vi "UpdateCtrlParams.vi"(6 "Ignore Update? (F)":bool, 8 "error in (no error)":errorcluster, 9 "Ts [s]":dbl caption="FPGA Ctrl Loop \nTime (Ts) [s]", 10 "Controller Gains":T2={"Z-direction"={"Kp"=1.0, "Ki"=50.0, "fLPF"=0.0}, "ThX-direction"={"Kp"=1.0, "Ki"=0.0, "fLPF"=0.0}, "ThY-direction"={"Kp"=1.0, "Ki"=0.0, "fLPF"=0.0}, "Bow-direction"={"Kp"=1.0, "Ki"=0.0, "fLPF"=0.0}, "Tor-direction"={"Kp"=0.0, "Ki"=0.0, "fLPF"=0.0}}, 11 "FPGA VI Reference In":T1) -> (0 "error out":errorcluster, 3 "FPGA VI ReferenceOut":T1)   [LabVIEW 2020, in "FPGAcontrolIO.lvlib"]
doc: "Update FPGA controller parameters"
uses:
  FPGAcontrolIO.lvlib
  PC/Controller/TypeDefs/ControllerGains_UI.ctl
  PC/Controller/TypeDefs/ControllerGains_IndAxis.ctl
  FPGA/Components/FPGA TypeDefs/FPGA_Ref_TypeDef.ctl
  PC/Components/Controller/TypeDefs/LPF params.ctl
  <vilib>/Utility/error.llb/Error Cluster From Error Code.vi
  <vilib>/rvi/errors/niLvFpgaAdjustHostInterfaceError.vi
  <vilib>/rvi/interface/nirviReadWriteControl/nirviReadWriteControl.xnode
  PC/Components/Controller/PC-RT_Controller.lvlib
  NiFpgaLv.dll
  <vilib>/rvi/interface/Simulation/niFpgaSimulationCallBeginRW.vi
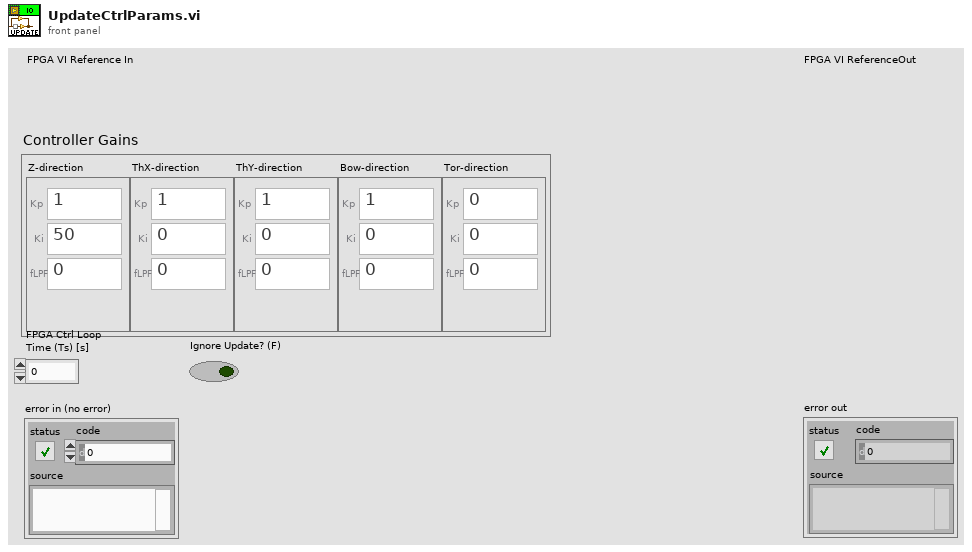
[diagram p1: front panel]
types:
  T1 = typedef "FPGA_Ref_TypeDef.ctl" = refnum<k20>
  T2 = typedef "ControllerGains_UI.ctl" = cluster{"Z-direction":T3, "ThX-direction":T3, "ThY-direction":T3, "Bow-direction":T3, "Tor-direction":T3}
  T3 = typedef "ControllerGains_IndAxis.ctl" = cluster{"Kp":dbl, "Ki":dbl, "fLPF":dbl}
  T4 = typedef "PC-RT_Controller.lvlib/LPF params.ctl" = cluster{"f_LPF [Hz]":dbl, "zeta":dbl}
  T5 = typedef "PC-RT_Controller.lvlib/TF_model.ctl" = cluster{"Numerator":dbl[], "Denominator":dbl[], "Sampling Time (Ts) [sec]":dbl}
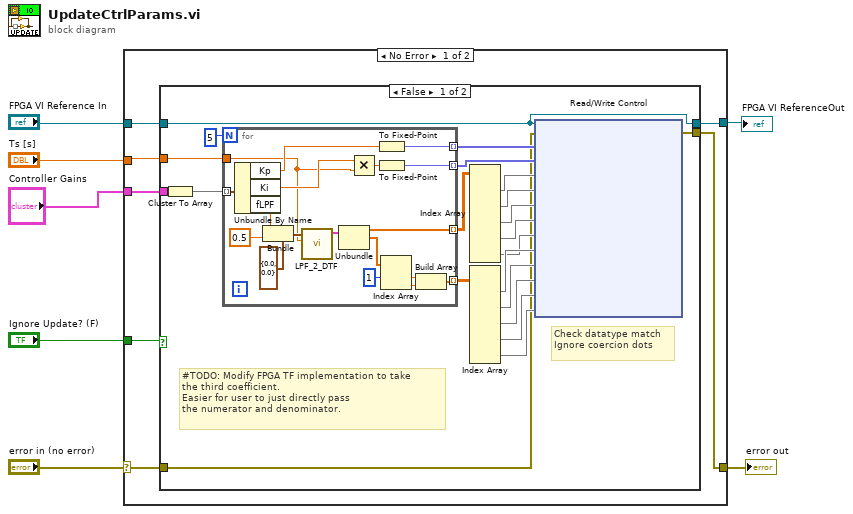
[diagram p0: block diagram]
diagram:
  n1 = case shown="No Error" "error in (no error)" {
    selector: "error in (no error)" -> [w12 w57]
    tunnel: [w11 w57] -> w6
    tunnel: "FPGA VI Reference In" -> [w9 w56]
    tunnel: "Controller Gains" -> [w14 _]
    tunnel: "Ts [s]" -> [w13 _]
    tunnel: "Ignore Update? (F)" -> [w10 _]
    tunnel: [w8 w56] -> w1
    frame No Error {
      n2 = case shown="False" w10 {
        tunnel: w9 -> [w15 w55]
        tunnel: w14 -> [w19 _]
        tunnel: w13 -> [w18 _]
        tunnel: w12 -> [w17 w54]
        tunnel: [w16 w54] -> w11
        tunnel: [w15 w55] -> w8
        frame False {
          # "#TODO: Modify FPGA TF implementation to take \nthe third coefficient. \nEasier for user to just directly pass \nthe numerator and denominator."
          # "Check datatype match\nIgnore coercion dots"
          n3 = Cluster To Array(cluster=w19) -> (array=w32:T3[])
          n4 = for {
            N: 5 -> [_]
            tunnel: [w53] -> w34 mode=indexing
            tunnel: [w52] -> w35 mode=indexing
            tunnel: w32 -> [w51] mode=indexing
            tunnel: [w42] -> w27 mode=indexing
            tunnel: [w37] -> w26 mode=indexing
            tunnel: w18 -> [w36]
            n5 = Unbundle By Name(w51) -> ("Kp"=w50:dbl, "Ki"=w48:dbl, "fLPF"=w47:dbl)
            n6 = Bundle(cluster=T4 {"f_LPF [Hz]"=0.0, "zeta"=0.0} ("LPF params"), "f_LPF [Hz]"=w47, "zeta"=0.5 ("fLPF")) -> (w45:T4)
            n7 = call "LPF_2_DTF.vi"("Sampling Time [s]"=w36, "LPF params"=w45) -> ("TF model"=w43:T5)  [unwired: 8 in, 1 out]
            n8 = Unbundle(w43) -> ("Numerator"=w42:dbl[], "Denominator"=w41:dbl[])  [unwired: 1 out]
            n9 = Multiply(x=w48, y=w36) -> (x*y=w49:dbl)
            n10 = To Fixed-Point(number=w50) -> (fixed-point=w53:fxp<+,17,17>)  [unwired: 1 in]
            n11 = To Fixed-Point(number=w49) -> (fixed-point=w52:fxp<+,17,0>)  [unwired: 1 in]
            n12 = Index Array(array=w41, index #1=1 ("index")) -> (element #1=w39:dbl, element #2=w38:dbl)  [unwired: 1 in]
            n13 = Build Array(w39, w38) -> (w37:dbl[])
          }
          n14 = Index Array(array=w27) -> (element #1=w31:dbl[], element #2=w30:dbl[], element #3=w29:dbl[], element #4=w28:dbl[], element #5=w21:dbl[])  [unwired: 10 in]
          n15 = Index Array(array=w26) -> (element #1=w25:dbl[], element #2=w24:dbl[], element #3=w23:dbl[], element #4=w22:dbl[], element #5=w20:dbl[])  [unwired: 10 in]
          n16 = xnode "Read/Write Control"("FPGA VI Reference In"=w15, "error in"=w17, "Kp"=w34, "Ki*Ts"=w35, "Numerator (b0, b1, b2)"=w31, "Numerator (b0, b1, b2) 2"=w30, "Numerator (b0, b1, b2) 3"=w29, "Numerator (b0, b1, b2) 4"=w28, "Numerator (b0, b1, b2) 5"=w21, "Denominator (a1, a2)"=w25, "Denominator (a1, a2) 2"=w24, "Denominator (a1, a2) 3"=w23, "Denominator (a1, a2) 4"=w22, "Denominator (a1, a2) 5"=w20) -> ("error out"=w16:errorcluster)  [unwired: 1 out]
        }
        frame True {
        }
      }
    }
    frame Error {
    }
  }
  "error out" <- w6
  "FPGA VI ReferenceOut" <- w1
